vi "Check executables admin priviledges.vi"() -> (0 "error out":errorcluster, 3 "Exe not run as an administrator":bool)   [LabVIEW 2013]
uses:
  Typedefs/Which path.ctl
  <vilib>/Utility/config.llb/Read Key (Boolean).vi
  <vilib>/Utility/config.llb/Write Key (Boolean).vi
  <vilib>/Utility/config.llb/NI_LVConfig.lvlib
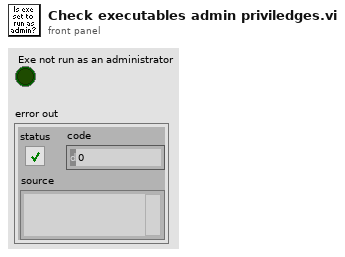
[diagram p1: front panel]
types:
  T1 = typedef "Which path.ctl" = enum16{"Configuration Files", "Calibration Files", "Images", "Setup.ini", "Loaded User profile.ini", "User's-Previous session.ini", "New user profile.ini", "Selected User profile.ini", "User profiles folder", "Power meter scaling.txt", "FOV Cal.ini"}
  T2 = typedef "NI_LVConfig.lvlib/Config Data RefNum.ctl" = refnum<k1>
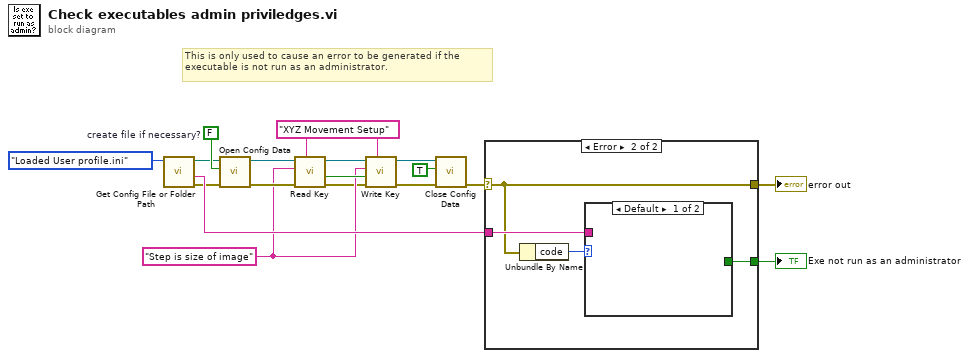
[diagram p0: block diagram]
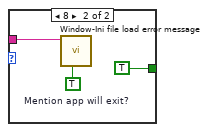
[diagram p3: hidden frame]
diagram:
  w4 = "Step is size of image" ("key")
  w5 = "XYZ Movement Setup" ("section")
  w17 = FALSE  # create file if necessary?
  # "This is only used to cause an error to be generated if the executable is not run as an administrator."
  n1 = call "Get Config File or Folder Path.vi"("Which file or folder?"=Which_path."Loaded User profile.ini" ("Which path?")) -> ("Error Out"=w13:errorcluster, "File/Folder name string"=w14:string, "File Path"=w12:path)  [unwired: 8 in]
  n2 = call <vilib>:"Open Config Data.vi"("error in (no error)"=w13, "create file if necessary (T)"=w17, "configuration file path"=w12) -> ("error out"=w11:errorcluster, "refnum"=w8:T2)  [unwired: 6 in, 1 out]
  n3 = call-poly <vilib>:"Read Key.vi"("section"=w5, "error in (no error)"=w11, "key"=w4, "refnum"=w8) -> ("error out"=w3:errorcluster, "value"=w6:bool, "refnum out"=w9:T2)  [unwired: 4 in, 1 out]
  n4 = call-poly <vilib>:"Write Key.vi"("section"=w5, "error in (no error)"=w3, "value"=w6, "key"=w4, "refnum"=w9) -> ("error out"=w10:errorcluster, "refnum out"=w7:T2)  [unwired: 4 in, 1 out]
  n5 = call <vilib>:"Close Config Data.vi"("error in (no error)"=w10, "write file if changed (T)"=TRUE ("write configuration file? (F)"), "refnum"=w7) -> ("error out"=w18:errorcluster)  [unwired: 7 in, 1 out]
  n6 = case shown="Error" w18 {
    selector: w18 -> [w19 w22]
    tunnel: w14 -> [_ w23]
    tunnel: [w19 w22] -> w1
    tunnel: [_ w20] -> w2
    frame No Error {
    }
    frame Error {
      n7 = Unbundle By Name(w22) -> ("code"=w21:i32)
      n8 = case shown="Default" w21 {
        tunnel: w23 -> [_ w26]
        tunnel: [_ TRUE] -> w20
        frame Default {
        }
        frame 8 {
          w25 = TRUE  # Mention app will exit?
          n9 = call "Window-Ini file load error message.vi"("Mention app will exit? (F)"=w25, "Message"=w26) -> ()  [unwired: 9 in, 1 out]
        }
      }
    }
  }
  "error out" <- w1
  "Exe not run as an administrator" <- w2
